vi "Vision Global.vi"() -> ()   [LabVIEW 2015]
panel:
  out "Vision Tracking":T1(array[cluster]) {"Normalized Rect"."Numeric 5" format="%#_2g"; "Normalized Rect"."Numeric 3" format="%#_2g"; "Normalized Rect"."Numeric 2" format="%#_2g"; "Normalized Rect"."Numeric" format="%#_2g"}
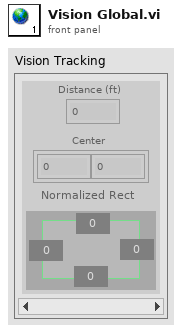
[diagram p1: front panel]
types:
  T1 = cluster{"Distance (ft)":dbl, "Center":cluster{dbl, dbl}, "Normalized Rect":cluster{"Numeric":dbl, "Numeric 2":dbl, "Numeric 3":dbl, "Numeric 5":dbl}}[]
diagram:
